vi "Rel to Abs Path.vi"(9 "Rel File Path":path, 11 "Base Path":path) -> (1 "Path":string, 3 "Path Out":path)   [LabVIEW 2010]
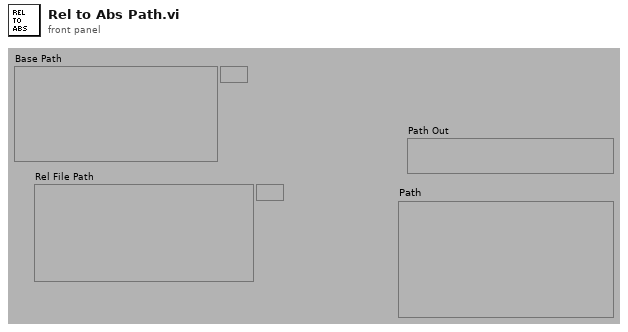
[diagram p1: front panel]
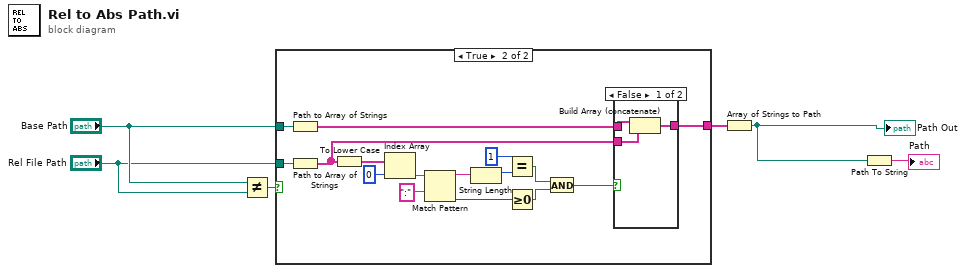
[diagram p0: block diagram]
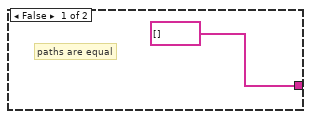
[diagram p2: hidden frame]
diagram:
  n1 = Not Equal?(x="Base Path", y="Rel File Path") -> (x != y?=w4:bool)
  n2 = case shown="True" w4 {
    tunnel: "Base Path" -> [_ w23]
    tunnel: "Rel File Path" -> [_ w22]
    tunnel: [string[] [] ("array of strings") w8] -> w3
    frame False {
      # "paths are equal"
    }
    frame True {
      n3 = Path to Array of Strings(0:w23) -> (2:w10:string[])  [unwired: 1 out]
      n4 = Path to Array of Strings(0:w22) -> (2:w9:string[])  [unwired: 1 out]
      n5 = To Lower Case(string=w9) -> (all lower case string=w21:string[])
      n6 = Index Array(array=w21, index=0) -> (element=w12:string)
      n7 = Match Pattern(string=w12, regular expression=":") -> (before substring=w18:string, offset past match=w15:i32)  [unwired: 1 in, 2 out]
      n8 = String Length(string=w18) -> (length=w17:i32)
      n9 = Equal?(x=1, y=w17) -> (x = y?=w13:bool)
      n10 = Greater Or Equal To 0?(x=w15) -> (x >= 0?=w14:bool)
      n11 = And(x=w13, y=w14) -> (x .and. y?=w11:bool)
      n12 = case shown="False" w11 {
        tunnel: w10 -> [w25 _]
        tunnel: w9 -> [w26 w27]
        tunnel: [w24 w27] -> w8
        frame False {
          n13 = Build Array (concatenate)(w25, w26) -> (w24:string[])
        }
        frame True {
        }
      }
    }
  }
  n14 = Array of Strings to Path(0:w3) -> (2:w2:path)  [unwired: 1 in]
  "Path Out" <- w2
  n15 = Path To String(path=w2) -> (string=→"Path":string)
